vi "Wait on Instrument String Response.vi"(8 "error in (no error)":errorcluster, 11 "Response Queue":T1) -> (0 "error out":errorcluster, 2 "Response":T2, 3 "message queue out":T1)   [LabVIEW 2018, in "Instrument Addon Engine.lvlib"]
uses:
  Instrument Addon Engine.lvlib
  Addon Shared/Types/Buffered RT Instrument Request.ctl
  <vilib>/NI/AMC/Message Queue.ctl
  <vilib>/NI/AMC/Message.ctl
  <vilib>/NI/Tools/Keyed Array/KeyedArray.ctl
  <vilib>/NI/AMC/Read Termination Message.vi
  <vilib>/NI/AMC/Create Single Message.vi
  <vilib>/NI/AMC/Globals.vi
  <vilib>/NI/AMC/AMC.lvlib
  Addon Shared/Instrument Addon Shared.lvlib
  <vilib>/NI/Tools/Keyed Array/Tools_KeyedArray.lvlib
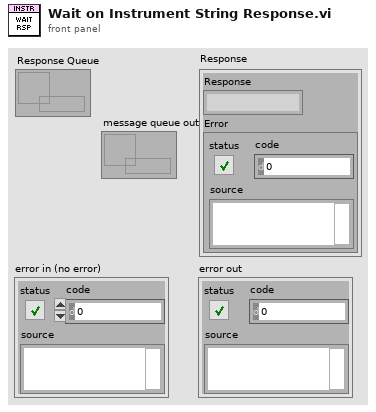
[diagram p1: front panel]
types:
  T1 = typedef "AMC.lvlib/Message Queue.ctl" = refnum<queue>
  T2 = typedef "Instrument Addon Shared.lvlib/Buffered RT Instrument Request.ctl" = cluster{"Response":string, "Error":errorcluster}
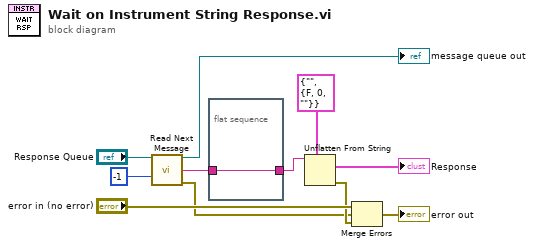
[diagram p0: block diagram]
diagram:
  n1 = call <vilib>:"Read Next Message.vi"("message queue in"="Response Queue", "timeout (1 ms)"=-1) -> ("message queue out"=→"message queue out":T1, "message value"=w10:string, "error out"=w2:errorcluster)  [unwired: 6 in, 5 out]
  n2 = flat-sequence {
    tunnel: [w12] -> w9
    tunnel: w10 -> [w12]
    frame #0 {
    }
  }
  n3 = Unflatten From String(type=T2 {"Response"="", "Error"={"status"=FALSE, "code"=0, "source"=""}}, binary string=w9) -> (value=→"Response":T2, error out=w3:errorcluster)  [unwired: 3 in, 1 out]
  n4 = Merge Errors("error in (no error)", w2, w3) -> (→"error out":errorcluster)
